vi "选择操作日志还是报警信息 (子VI).vi"(10 "搜索字符串":string(combo), 11 "Value":string) -> (2 "布尔":bool, 3 "功能":string)   [LabVIEW 2016, in "数据传输系统.lvlib"]
panel:
  out "子字符串;substring":string
  # "PolId=w01018,InfoId=i11001;BeginTime=20160801010522,EndTime=20160801085857"
  # "PolId=w01018,InfoId=i12001"
  # "PolId=w01018,InfoId=i13004"
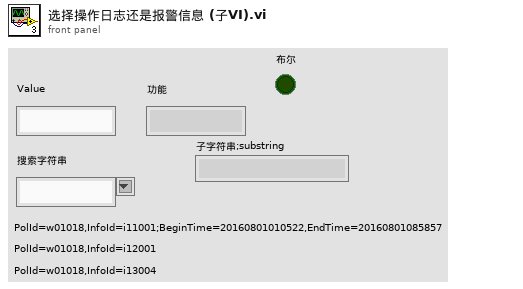
[diagram p1: front panel]
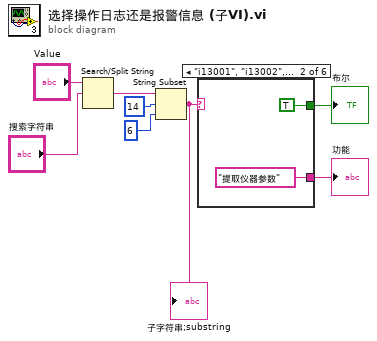
[diagram p0: block diagram]
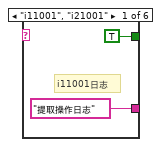
[diagram p2: hidden frame]
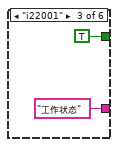
[diagram p3: hidden frame]
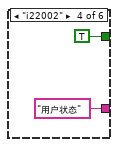
[diagram p4: hidden frame]
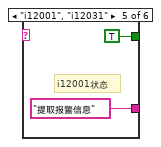
[diagram p5: hidden frame]
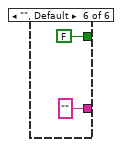
[diagram p6: hidden frame]
diagram:
  n1 = Search/Split String(string="Value", search string/char (-)="搜索字符串") -> (match + rest of string=w5:string)  [unwired: 1 in, 2 out]
  n2 = String Subset(string=w5, offset (0)=14 ("偏移量(0)"), length (rest)=6 ("长度（剩余）")) -> (substring=w2:string)
  "子字符串;substring" <- w2
  n3 = case shown="\"i13001\", \"i13002\", \"i13003\", \"i13004\", \"i13005\", \"i13006\", \"i13007\", \"i13008\", \"i13009\", \"i13010\", \"i13011\", \"i13012\", \"i13013\", \"i13014\", \"i13015\", \"i13016\", \"i13017\", \"i13101\", \"i13102\", \"i13103\", \"i13104\", \"i13105\", \"i13106\", \"i13107\", \"i13108\", \"i13109\", \"i13110\"" w2 {
    tunnel: ["提取操作日志" ("名称（未命名）") "提取仪器参数" ("名称（未命名）") "工作状态" ("名称（未命名）") "用户状态" ("名称（未命名）") "提取报警信息" ("名称（未命名）") "" ("名称（未命名）")] -> w8
    tunnel: [TRUE TRUE TRUE TRUE TRUE FALSE] -> w1
    frame "i11001", "i21001" {
      # "i11001日志"
    }
    frame "i13001", "i13002", "i13003", "i13004", "i13005", "i13006", "i13007", "i13008", "i13009", "i13010", "i13011", "i13012", "i13013", "i13014", "i13015", "i13016", "i13017", "i13101", "i13102", "i13103", "i13104", "i13105", "i13106", "i13107", "i13108", "i13109", "i13110" {
    }
    frame "i22001" {
    }
    frame "i22002" {
    }
    frame "i12001", "i12031" {
      # "i12001状态"
    }
    frame "", Default {
    }
  }
  "功能" <- w8
  "布尔" <- w1
